vi "CreateScanDefinitionMenu.vi"(0 "menu reference":refnum<k9>, 5 "error in (no error)":errorcluster) -> (19 "error out":errorcluster)   [LabVIEW 2020]
doc: "This VI creates menu entries for scan definition SubVIs."
panel:
  out "menu reference out":refnum<k9>
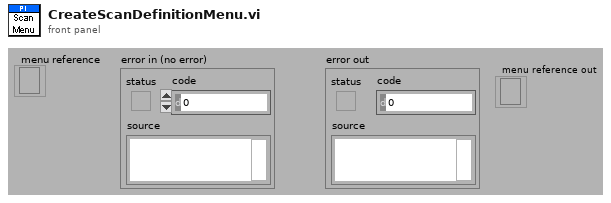
[diagram p1: front panel]
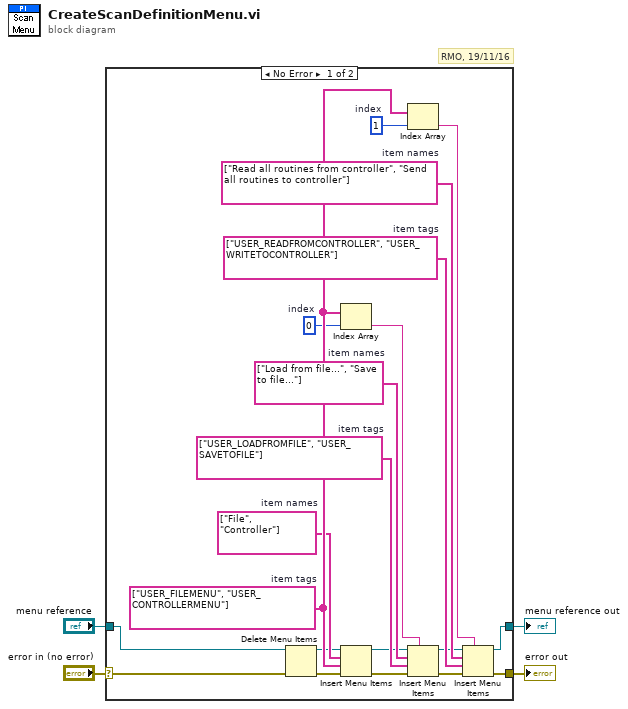
[diagram p0: block diagram]
diagram:
  # "RMO, 19/11/16"
  n1 = case shown="No Error" "error in (no error)" {
    selector: "error in (no error)" -> [w5 w26]
    tunnel: [w24 w26] -> w4
    tunnel: "menu reference" -> [w7 w25]
    tunnel: [w6 w25] -> w2
    frame No Error {
      w22 = string[] ["USER_READFROMCONTROLLER", "USER_WRITETOCONTROLLER"]  # item tags
      w20 = string[] ["Read all routines from controller", "Send all routines to controller"]  # item names
      w15 = string[] ["USER_LOADFROMFILE", "USER_SAVETOFILE"]  # item tags
      w14 = string[] ["Load from file...", "Save to file..."]  # item names
      w23 = string[] ["USER_FILEMENU", "USER_CONTROLLERMENU"]  # item tags
      w19 = string[] ["File", "Controller"]  # item names
      w18 = 1  # index
      w16 = 0  # index
      n2 = Delete Menu Items(6:w5, 9:w7) -> (0:w9:errorcluster, 3:w8:refnum<k9>)  [unwired: 2 out]
      n3 = Index Array(array=w23, index=w16) -> (element=w17:string)
      n4 = Insert Menu Items(6:w9, 7:w23, 8:w19, 9:w8) -> (0:w10:errorcluster, 3:w12:refnum<k9>)  [unwired: 3 out]
      n5 = Index Array(array=w23, index=w18) -> (element=w21:string)
      n6 = Insert Menu Items(5:w17, 6:w10, 7:w15, 8:w14, 9:w12) -> (0:w11:errorcluster, 3:w13:refnum<k9>)  [unwired: 2 out]
      n7 = Insert Menu Items(5:w21, 6:w11, 7:w22, 8:w20, 9:w13) -> (0:w24:errorcluster, 3:w6:refnum<k9>)  [unwired: 2 out]
    }
    frame Error {
    }
  }
  "error out" <- w4
  "menu reference out" <- w2
